vi "stage and voice coil synchronization Lin V3.vi"() -> ()   [LabVIEW 2020]
uses:
  <vilib>/DAQmx/write.llb/DAQmx Write (Analog 2D DBL NChan NSamp).vi
  <vilib>/Analysis/1siggen.llb/Ramp Pattern by Delta.vi
  <vilib>/DAQmx/create/channels.llb/DAQmx Create Channel (AO-Voltage-Basic).vi
  <vilib>/DAQmx/create/channels.llb/DAQmx Create Channel (CO-Pulse Generation-Frequency).vi
  <vilib>/DAQmx/configure/timing.llb/DAQmx Timing (Implicit).vi
  <vilib>/DAQmx/configure/timing.llb/DAQmx Timing (Sample Clock).vi
  <vilib>/DAQmx/miscellaneous.llb/DAQmx Fill In Error Info.vi
  <vilib>/Analysis/NI_AALBase.lvlib
  <vilib>/measure/NI_MABase.lvlib
panel:
  out "Waveform Graph 2":waveform(dbl)(graph)
  in  "y":bool
  out "error out":errorcluster
  out "number of samples written per channel":u32=4000
  out "samples":i32=4000
  out "Waveform Graph":waveform(dbl)[](graph)=[{"t0"=timestamp(0 s since 1904-01-01), "dt"=0.001, "Y"=array[4000 elements]}, {"t0"=timestamp(0 s since 1904-01-01), "dt"=0.001, "Y"=array[4000 elements]}]
  out "Number of slices":dbl=4000.0
  in  "End position (mm)":dbl=4.0
  out "Total Z thickness (mm)":dbl=3.999
  in  "Z slice width (mm)":dbl=0.001
  in  "Start position(mm)":dbl=0.001
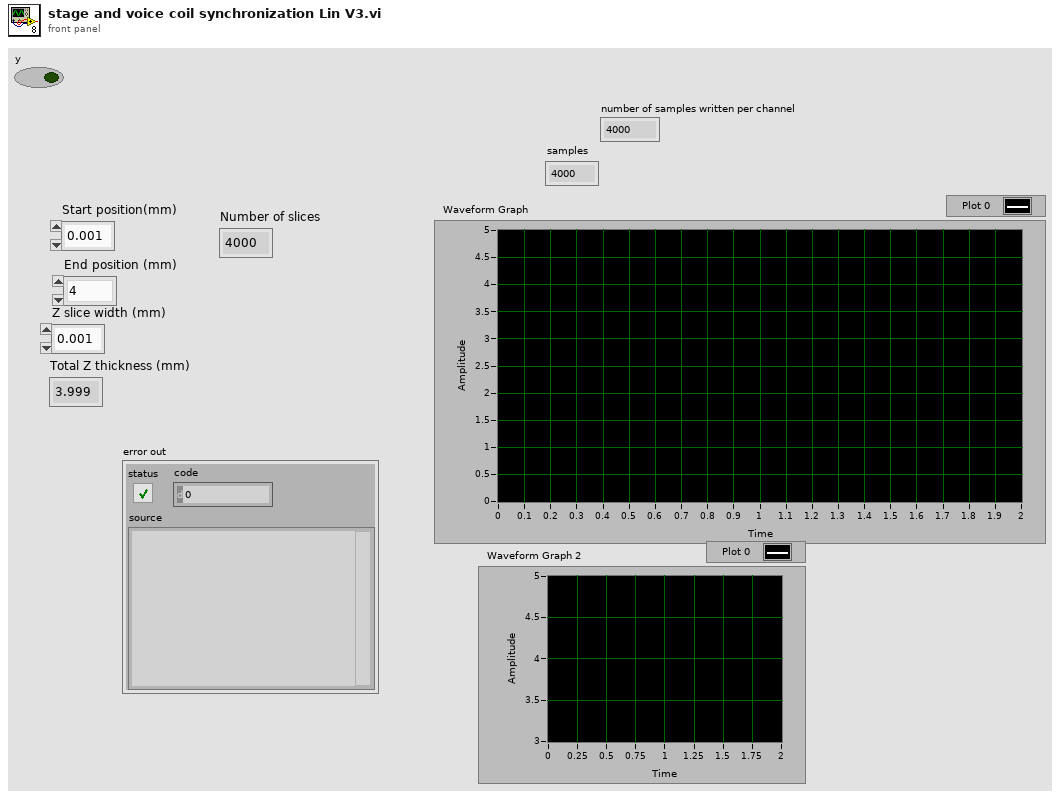
[diagram p1: front panel]
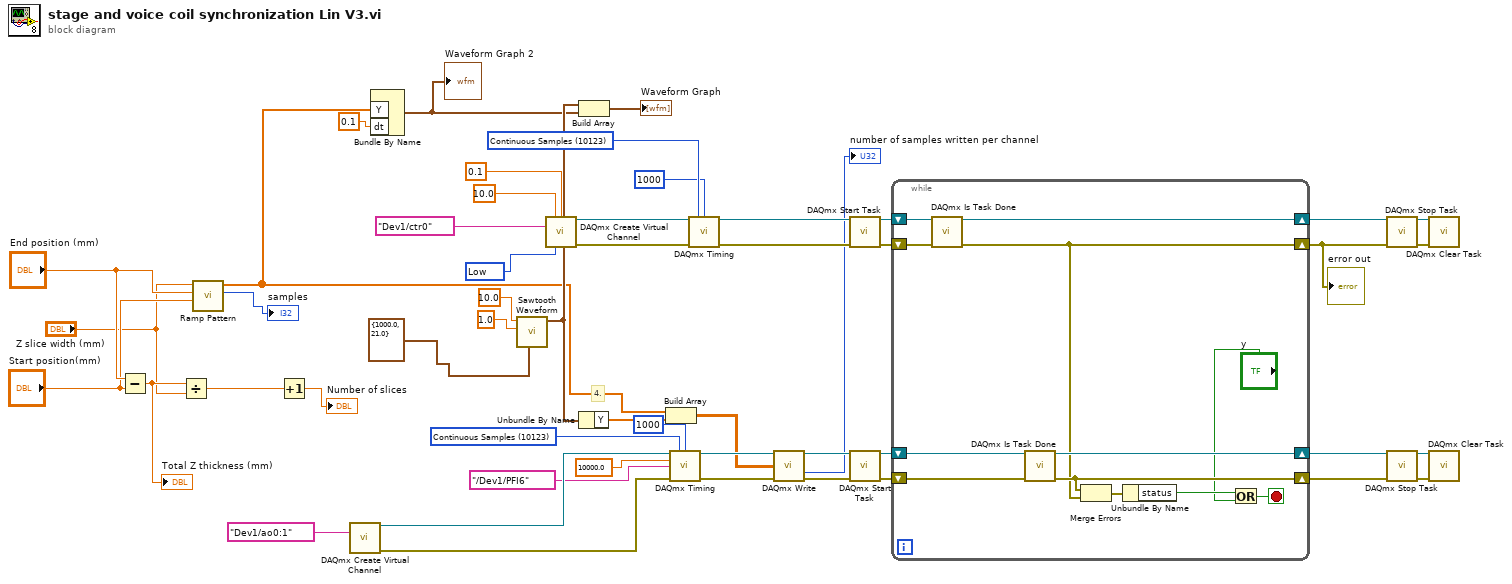
[diagram p0: block diagram]
diagram:
  w31 = 10214 items=["High"=10192, "Low"=10214] ("idle state")
  w33 = 10123 items=["Finite Samples"=10178, "Continuous Samples"=10123, "Hardware Timed Single Point"=12522] ("sample mode")
  w39 = 10123 items=["Finite Samples"=10178, "Continuous Samples"=10123, "Hardware Timed Single Point"=12522] ("sample mode")
  # "4."
  n1 = Subtract(x="End position (mm)", y="Start position(mm)") -> (x-y=w51:dbl)
  "Total Z thickness (mm)" <- w51
  n2 = Divide(x=w51, y="Z slice width (mm)") -> (x/y=w15:dbl)
  n3 = call-poly <vilib>:"Ramp Pattern.vi"("start"="Start position(mm)", "end"="End position (mm)", "delta"="Z slice width (mm)") -> ("samples"=→"samples":i32, "Ramp Pattern"=w13:dbl[])  [unwired: 6 in, 1 out]
  n4 = Increment(x=w15) -> (x+1=→"Number of slices":dbl)
  n5 = call-poly <vilib>:"DAQmx Create Virtual Channel.vi"("physical channels"=tag "Dev1/ao0:1") -> ("task out"=w41:refnum<k21>, "error out"=w40:errorcluster)  [unwired: 13 in]
  n6 = Bundle By Name("Y"=w13, "dt"=0.1) -> (w2:waveform(dbl))  [unwired: 1 in]
  "Waveform Graph 2" <- w2
  n7 = call <vilib>:"Sawtooth Waveform.vi"("sampling info"=cluster{"Fs":dbl, "#s":dbl} {"Fs"=1000.0, "#s"=21.0}, "amplitude"=1.0, "frequency"=10.0) -> ("signal out"=w14:waveform(dbl))  [unwired: 7 in, 1 out]
  n8 = call-poly <vilib>:"DAQmx Create Virtual Channel.vi"("frequency"=10.0, "duty cycle"=0.1, "counter"=tag "Dev1/ctr0", "idle state"=w31) -> ("task out"=w36:refnum<k21>, "error out"=w35:errorcluster)  [unwired: 10 in]
  n9 = Build Array(w14, w2) -> (→"Waveform Graph":waveform(dbl)[])
  n10 = Unbundle By Name(w14) -> ("Y"=w12:dbl[])
  n11 = Build Array(w13, w12) -> (w11:dbl[][])
  n12 = call-poly <vilib>:"DAQmx Timing.vi"("task/channels in"=w41, "sample mode"=w39, "samples per channel"=1000, "rate"=10000.0, "source"=tag "/Dev1/PFI6", "error in"=w40) -> ("task out"=w26:refnum<k21>, "error out"=w27:errorcluster)  [unwired: 8 in]
  n13 = call-poly <vilib>:"DAQmx Timing.vi"("task/channels in"=w36, "sample mode"=w33, "samples per channel"=1000, "error in"=w35) -> ("task out"=w29:refnum<k21>, "error out"=w28:errorcluster)  [unwired: 10 in]
  n14 = call-poly <vilib>:"DAQmx Write.vi"("task/channels in"=w26, "data"=w11, "error in"=w27) -> ("task out"=w10:refnum<k21>, "number of samples written per channel"=→"number of samples written per channel":u32, "error out"=w9:errorcluster)  [unwired: 10 in]
  n15 = call <vilib>:"DAQmx Start Task.vi"("task/channels in"=w29, "error in"=w28) -> ("task out"=w38:refnum<k21>, "error out"=w37:errorcluster)  [unwired: 12 in]
  n16 = call <vilib>:"DAQmx Start Task.vi"("task/channels in"=w10, "error in"=w9) -> ("task out"=w8:refnum<k21>, "error out"=w7:errorcluster)  [unwired: 12 in]
  n17 = while {
    shift-right: [w60] -> w43
    shift-left: w8 -> [w59]
    shift-right: [w61] -> w49
    shift-left: w38 -> [w63]
    shift-right: [w54] -> w47
    shift-left: w37 -> [w62]
    shift-right: [w55] -> w45
    shift-left: w7 -> [w58]
    stop <- w56 stop-if-true
    n18 = call <vilib>:"DAQmx Is Task Done.vi"("task/channels in"=w63, "error in"=w62) -> ("task out"=w61:refnum<k21>, "error out"=w54:errorcluster)  [unwired: 11 in, 1 out]
    n19 = call <vilib>:"DAQmx Is Task Done.vi"("task/channels in"=w59, "error in"=w58) -> ("task out"=w60:refnum<k21>, "error out"=w55:errorcluster)  [unwired: 11 in, 1 out]
    n20 = Merge Errors(w55, w54) -> (w53:errorcluster)
    n21 = Unbundle By Name(w53) -> ("status"=w57:bool)
    n22 = Or(x=w57, y="y") -> (x .or. y?=w56:bool)
  }
  "error out" <- w47
  n23 = call <vilib>:"DAQmx Stop Task.vi"("task/channels in"=w49, "error in"=w47) -> ("task out"=w48:refnum<k21>, "error out"=w46:errorcluster)  [unwired: 12 in]
  n24 = call <vilib>:"DAQmx Stop Task.vi"("task/channels in"=w43, "error in"=w45) -> ("task out"=w42:refnum<k21>, "error out"=w44:errorcluster)  [unwired: 12 in]
  n25 = call <vilib>:"DAQmx Clear Task.vi"("task in"=w48, "error in"=w46) -> ()  [unwired: 13 in, 1 out]
  n26 = call <vilib>:"DAQmx Clear Task.vi"("task in"=w42, "error in"=w44) -> ()  [unwired: 13 in, 1 out]
